vi "2 Think.vi"() -> ()   [LabVIEW 2011]
doc: "The Think VI performs the logic to determine which setpoints to send to the boat. Within the Think VI, a variety of systems take the boat information and output sail and rudder setpoints. The Think VI contains the arbiter VI which contains the logic used to determine which setpoints will ultimately be sent to the boat.\n\nWithin the Think VI, 5 systems are considered, in order of inherent priority:\n-Manual Override\n-Don't Flip\n-Staying out of/getting out of Irons\n-Getting to the goal\n-Default (such that there is always something being sent to the boat)"
uses:
  2 Typedefs/setpoints to boat.ctl
  2 Typedefs/sail setpt.ctl
  2 Typedefs/rudder angle.ctl
  2 Typedefs/setpoints to arbiter.ctl
  2 Globals/2 Global.vi
panel:
  out "Default Setpoints":T1
  out "Get to Goal Setpoints":T1
  out "Get Out of Irons Setpoints":T1
  out "Don't Flip Setpoints":T1
  out "Override Setpoints":T1
  out "Final Setpoints":T2
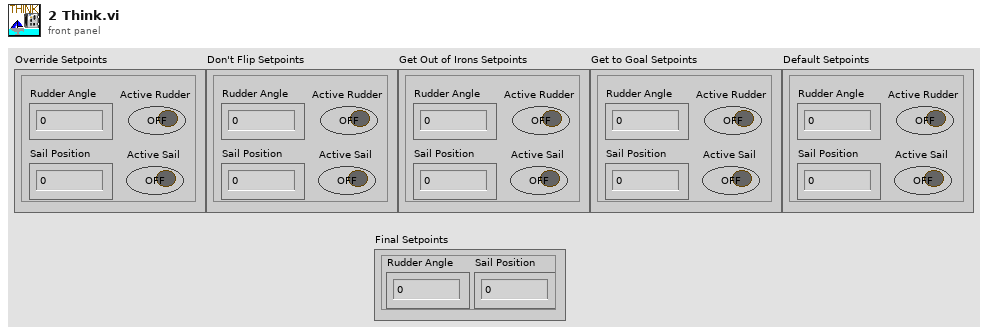
[diagram p1: front panel]
types:
  T1 = typedef "setpoints to arbiter.ctl" = cluster{"Rudder Angle":dbl, "Sail Position":dbl, "Active Rudder":bool, "Active Sail":bool}
  T2 = typedef "setpoints to boat.ctl" = cluster{"Sail Position":T3, "Rudder Angle":T4}
  T3 = typedef "sail setpt.ctl" = dbl
  T4 = typedef "rudder angle.ctl" = dbl
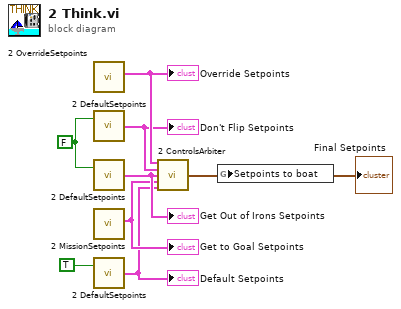
[diagram p0: block diagram]
diagram:
  w4 = FALSE
  n1 = call "2 OverrideSetpoints.vi"() -> ("Setpoints Out"=w7:T1)  [unwired: 11 in]
  "Override Setpoints" <- w7
  n2 = call "2 DefaultSetpoints.vi"("Use Defaults"=w4) -> ("Setpoint Cluster"=w6:T1)  [unwired: 1 in]
  "Don't Flip Setpoints" <- w6
  n3 = call "2 DefaultSetpoints.vi"("Use Defaults"=w4) -> ("Setpoint Cluster"=w3:T1)  [unwired: 1 in]
  "Get Out of Irons Setpoints" <- w3
  n4 = call "2 MissionSetpoints.vi"() -> ("Setpoints Out"=w2:T1)  [unwired: 11 in]
  "Get to Goal Setpoints" <- w2
  n5 = call "2 DefaultSetpoints.vi"("Use Defaults"=TRUE) -> ("Setpoint Cluster"=w1:T1)  [unwired: 1 in]
  "Default Setpoints" <- w1
  n6 = call "2 ControlsArbiter.vi"("Manual Setpoints"=w7, "Dont Flip Setpoints"=w6, "Get out of Irons Setpoints"=w3, "Get to Goal Setpoints"=w2, "Default Setpoints"=w1) -> ("Final Setpoints"=w8:T2)  [unwired: 10 in]
  "Final Setpoints" <- w8
  n7 = global write "2 Global.vi" "Setpoints to boat"(w8) -> ()
